vi "Get configuration chain.vi"(8 "error in (no error)":errorcluster, 11 "RetigaBase in":refnum<class "Retiga.lvclass">) -> (0 "error out":errorcluster, 1 "class name":string[](array[string]), 2 "configuration chain":variant[](array[variant]), 3 "RetigaBase out":refnum<class "Retiga.lvclass">)   [LabVIEW 2012, in "Retiga.lvclass"]
doc: "Returns an array of variants containing the configuration clusters of each class in the inheritance chain (lowest child class first), together with an array of all class names in the inheritance chain.\n\nFor classes without configuration cluster, the configuration chain contains empty variants."
uses:
  Retiga.lvclass
  <vilib>/Distrio/Murmex/Murmex/Murmex.lvclass
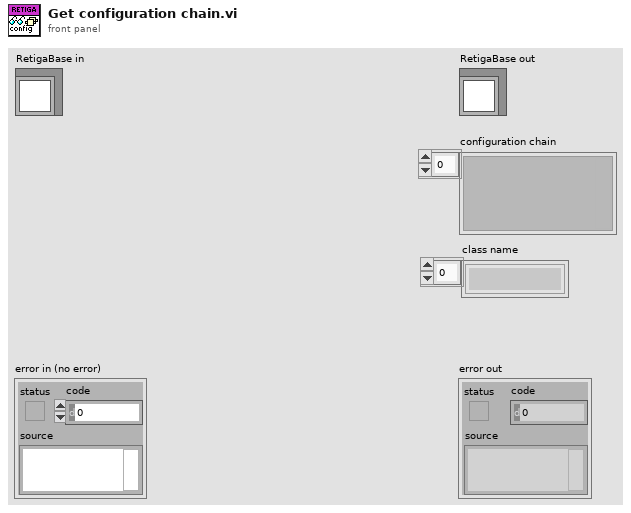
[diagram p1: front panel]
types:
  T1 = typedef "Retiga.lvclass/configuration.ctl" = cluster{"temperature":dbl, "stage component":string, "micron equivalent of pixel":dbl[unit], "max x pixel displacement":dbl, "min x pixel displacement":dbl, "max pixel discrepancy":dbl, "max y pixel displacement":dbl, "min y pixel displacement":dbl, "brightness threshold":sgl}
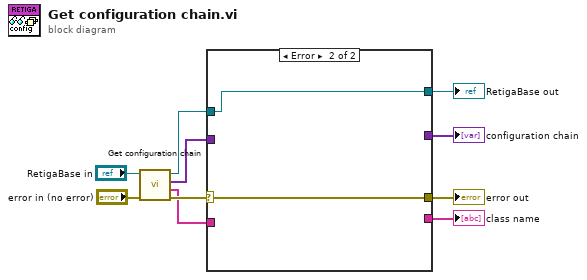
[diagram p0: block diagram]
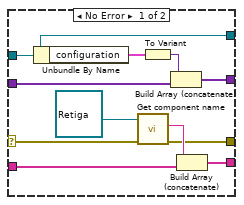
[diagram p2: hidden frame]
diagram:
  n1 = call-parent "Get configuration chain.vi"("error in (no error)"="error in (no error)", "MurmexBase in"="RetigaBase in") -> ("error out"=w8:errorcluster, "class name"=w5:string[], "configuration chain"=w6:variant[], "MurmexBase out"=w7:refnum<class "Retiga.lvclass">)  [unwired: 6 in]
  n2 = case shown="Error" w8 {
    selector: w8 -> [w19 w22]
    tunnel: w7 -> [w13 w23]
    tunnel: w6 -> [w18 _]
    tunnel: w5 -> [w17 _]
    tunnel: [w13 w23] -> w4
    tunnel: [w16 _] -> w3
    tunnel: [w15 w22] -> w2
    tunnel: [w14 _] -> w1
    frame No Error {
      n3 = Unbundle By Name(w13) -> ("configuration"=w12:T1)
      n4 = call <vilib>:"Get component name.vi"("error in (no error)"=w19, "Murmex in"=refnum<class "Retiga.lvclass"> refnum ("RetigaBase in")) -> ("error out"=w15:errorcluster, "component name"=w21:string)  [unwired: 7 in, 1 out]
      n5 = To Variant(anything=w12) -> (Variant=w20:variant)
      n6 = Build Array (concatenate)(w20, w18) -> (w16:variant[])
      n7 = Build Array (concatenate)(w21, w17) -> (w14:string[])
    }
    frame Error {
    }
  }
  "error out" <- w2
  "RetigaBase out" <- w4
  "configuration chain" <- w3
  "class name" <- w1
